vi "voltageScan.vi"() -> ()   [LabVIEW 2016]
uses:
  <vilib>/Utility/file.llb/Write Delimited Spreadsheet (DBL).vi
panel:
  in  "freq(MHz)":dbl=1.367
  out "voltnow":dbl
  out "OK？":bool
  out "Array":dbl[][](array[numeric])
  in  "sens":dbl=0.1284
  in  "osc in 2":refnum<visa-resource-name>
  in  "measure times":i16=8
  in  "volt step":dbl=0.5
  in  "end volt":dbl=7.0
  in  "start volt":dbl=2.0
  in  "HIFU port":u32=12321
  in  "HIFU ip":string="192.168.1.81"
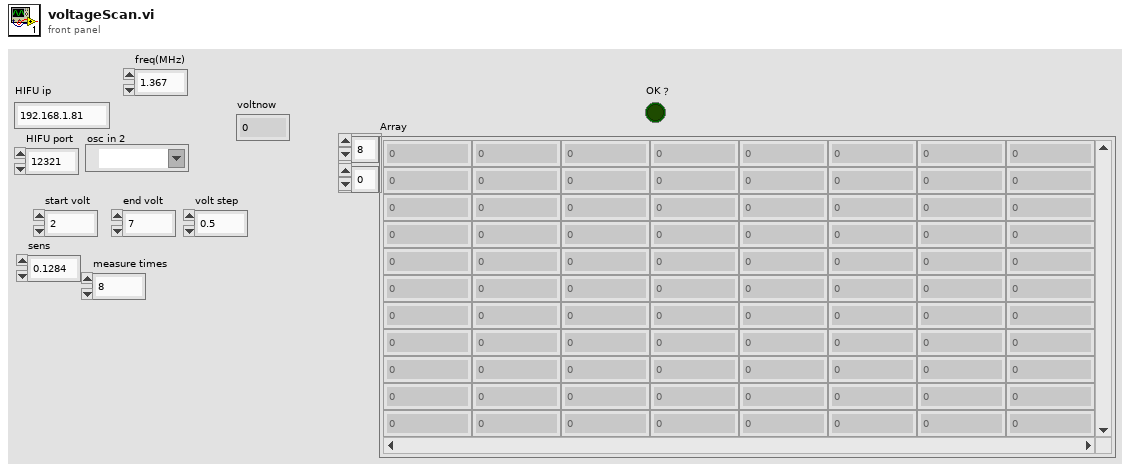
[diagram p1: front panel]
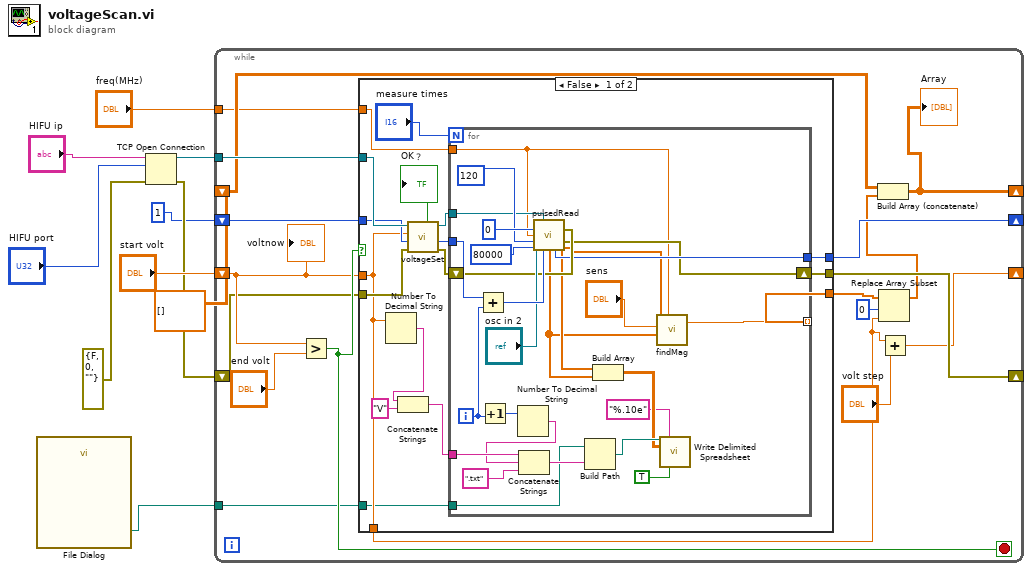
[diagram p0: block diagram]
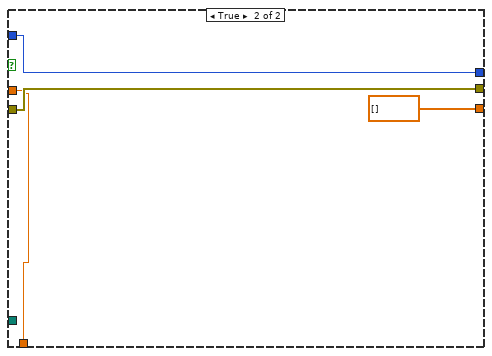
[diagram p2: hidden frame]
diagram:
  n1 = call "File Dialog"() -> ("selected path"=w1:path)  [unwired: 12 in, 3 out]
  n2 = TCP Open Connection(address="HIFU ip", remote port or service name="HIFU port", error in (no error)=errorcluster {"status"=FALSE, "code"=0, "source"=""} ("error out")) -> (connection ID=w7:refnum<k5>, error out=w5:errorcluster)  [unwired: 2 in]
  n3 = while {
    shift-right: [w18] -> _
    shift-left: "start volt" -> [w26]
    tunnel: w7 -> [w25]
    shift-right: [w20] -> _
    shift-left: w5 -> [w24]
    shift-right: [w22] -> _
    shift-left: 1 -> [w23]
    shift-right: [w17] -> _
    shift-left: dbl[][] [] -> [w21]
    tunnel: "freq(MHz)" -> [w12]
    tunnel: w1 -> [w11]
    stop <- w27 stop-if-true
    n4 = Greater?(x=w26, y="end volt") -> (0:w27:bool)
    n5 = case shown="False" w27 {
      tunnel: w26 -> [w33 w72]
      tunnel: w25 -> [w44 _]
      tunnel: w24 -> [w43 w74]
      tunnel: w23 -> [w42 w75]
      tunnel: [w38 w75] -> w22
      tunnel: [w37 dbl[] []] -> w15
      tunnel: [w33 w72] -> w14
      tunnel: [w36 w74] -> w20
      tunnel: w12 -> [w34 _]
      tunnel: w11 -> [w29 _]
      frame False {
        n6 = Number To Decimal String(number=w33) -> (decimal integer string=w32:string)  [unwired: 1 in]
        n7 = Concatenate Strings(w32, "V" ("string")) -> (w30:string)
        n8 = call "voltageSet.vi"("error in (no error)"=w43, "SEQ in"=w42, "Voltage"=w33, "connection ID"=w44) -> ("error out"=w39:errorcluster, "SEQ out"=w41:u32, "OK？"=→"OK？":bool, "connection ID out"=w40:refnum<k5>)
        n9 = for {
          N: "measure times" -> [_]
          tunnel: w41 -> [w68]
          tunnel: w40 -> [w65]
          tunnel: [w63] -> w38
          shift-right: [w62] -> w36
          shift-left: w39 -> [w64]
          tunnel: [w60] -> w37 mode=indexing
          tunnel: w34 -> [w59]
          tunnel: w30 -> [w54]
          tunnel: w29 -> [w50]
          i -> [w56]
          n10 = Add(x=w68, y=w56) -> (x+y=w67:u32)
          n11 = Increment(x=w56) -> (x+1=w55:i32)
          n12 = Number To Decimal String(number=w55) -> (decimal integer string=w53:string)  [unwired: 1 in]
          n13 = Concatenate Strings(w54, w53, ".txt" ("string")) -> (w51:string)
          n14 = call "pulsedRead.vi"("osc in"="osc in 2", "connection ID"=w65, "channel"=u8 0, "error in (no error)"=w64, "freq (MHz)"=w59, "cycles"=u64 120, "points"=u64 80000, "SEQ IN"=w67) -> ("error out"=w62:errorcluster, "voltage"=w57:dbl[], "SEQ OUT"=w63:u32, "time"=w58:dbl[])  [unwired: 2 in, 2 out]
          n15 = Build Path(base path=w50, name or relative path=w51) -> (appended path=w49:path)
          n16 = Build Array(w58, w57) -> (w48:dbl[][])
          n17 = call "findMag.vi"("times"=w58, "sens"="sens", "voltages"=w57, "freq"=w59) -> ("magfound"=w60:dbl)  [unwired: 1 in, 1 out]
          n18 = call-poly <vilib>:"Write Delimited Spreadsheet.vi"("file path (dialog if empty)"=w49, "format (%.3f)"="%.10e", "2D data"=w48, "transpose? (no:F)"=TRUE) -> ()  [unwired: 10 in, 2 out]
        }
      }
      frame True {
      }
    }
    n19 = Replace Array Subset(array=w15, new element=w14, index=0) -> (w13:dbl[])
    n20 = Build Array (concatenate)(w21, w13) -> (w17:dbl[][])
    "Array" <- w17
    n21 = Add(x=w14, y="volt step") -> (x+y=w18:dbl)
    "voltnow" <- w26
  }
